vi "UHR-Fleezers Control (host) - 11.9c.vi"() -> ()   [LabVIEW 2014] (continued)
          tunnel: [w2795] -> w2786
          tunnel: w2792 -> [w2812]
          tunnel: w2791 -> [w2811]
          tunnel: [w2809] -> w2790
          tunnel: w2789 -> [w2810]
          tunnel: [w2808] -> w2788
          tunnel: [w2807] -> w2787
          tunnel: w2786 -> [w2807]
          tunnel: w2790 -> [w2816]
          tunnel: w2788 -> [w2815]
          tunnel: w2787 -> [w2814]
          frame #0 {
            n1958 = call "Read Stage Position.vi"("error in"=w2805, "VISA resource name in"=w2797) -> ("Current Position"=w2795:cluster{dbl, dbl, dbl}, "error out"=w2798:errorcluster, "VISA resource name out"=w2796:refnum<visa-resource-name>)  [unwired: 1 out]
            "Current Position" <- w2795
            n1959 = local write "Stage Control Serial Error"(w2798) -> ()
            n1960 = Unbundle(w2795) -> (w2802:dbl, w2804:dbl, w2800:dbl)
            n1961 = Add(x=w2804, y="Y change (mm)") -> (x+y=w2801:dbl)
            n1962 = Bundle(w2802, w2801, w2800) -> (w2799:cluster{dbl, dbl, dbl})  [unwired: 1 in]
          }
          frame #1 {
            # "move to new position and start saving"
            n1963 = local write "Stage Moving"(TRUE ("Stage Moving")) -> ()
            n1964 = local write "Start Saving"(TRUE ("Start Saving")) -> ()
            n1965 = call "Set Stage Position.vi"("Position"=w2812, "error in"=w2811, "VISA resource name in"=w2810) -> ("error out"=w2808:errorcluster, "VISA resource name out"=w2809:refnum<visa-resource-name>)  [unwired: 1 out]
          }
          frame #2 {
            # "go back to start"
            n1966 = call "Set Stage Position.vi"("Position"=w2814, "error in"=w2815, "VISA resource name in"=w2816) -> ()  [unwired: 3 out]
          }
          frame #3 {
            # "stop saving"
            n1967 = local write "Stop Saving"(TRUE ("Stop Saving")) -> ()
            n1968 = local write "Stage Moving"(FALSE ("Stage Moving")) -> ()
          }
        }
      }
      event "Move to Position 1", "Move to Position 2", "Move to Position 3", "Move to Position 4", "Move to Position 5", "Lower Ch. Cap.": Value Change {
        n1969 = event-data() -> ()  [unwired: 1 in, 5 out]
        n1970 = Or(x="Move to Position 5", y="Lower Ch. Cap.") -> (x .or. y?=w2822:bool)
        n1971 = Build Array("Move to Position 1", "Move to Position 2", "Move to Position 3", "Move to Position 4", w2822) -> (w2825:bool[])
        n1972 = Boolean Array To Number(Boolean array=w2825) -> (number=w2824:u32)
        n1973 = Logarithm Base 2(1:w2824) -> (0:w2823:dbl)
        n1974 = flat-sequence {
          tunnel: w2823 -> [w2834]
          tunnel: w2820 -> [w2832]
          tunnel: w2819 -> [w2831]
          frame #0 {
            n1975 = local read "Saved Stage Positions"() -> (w2842:dbl[][])
            n1976 = Array Subset(array=w2842, index (row)=w2834, length (row)=1 ("length"), index (col)=1 ("index"), length (col)=3 ("length")) -> (w2839:dbl[][])
            n1977 = Reshape Array(w2839, 3 ("dimension size")) -> (w2837:dbl[])
            n1978 = Array To Cluster(array=w2837) -> (cluster=w2836:cluster{"[0]":dbl, "[1]":dbl, "[2]":dbl})
            n1979 = call "Set Stage Position.vi"("Position"=w2836, "error in"=w2831, "VISA resource name in"=w2832) -> ("error out"=w2835:errorcluster)  [unwired: 2 out]
            n1980 = local write "Stage Moving"(TRUE ("Stage Moving")) -> ()
            n1981 = local write "Stage Control Serial Error"(w2835) -> ()
          }
          frame #1 {
            n1982 = local write "Stage Moving"(FALSE ("Stage Moving")) -> ()
            n1983 = call <vilib>:"Beep.vi"() -> ()  [unwired: 3 in, 9 out]
          }
        }
      }
      event "Set Current\nPos to 0,0,0": Value Change {
        # "DH is \"Define Home\""
        n1984 = event-data() -> ()  [unwired: 1 in, 6 out]
        n1985 = local write "Set Current\nPos to 0,0,0"(FALSE ("Set Current\nPos to 0,0,0")) -> ()
        n1986 = Concatenate Strings("1DH" ("string"), ";" ("string"), "2DH" ("string"), ";" ("string"), "3DH" ("string"), "\r") -> (w2850:string)
        n1987 = call-poly "VISA Configure Serial Port"("VISA resource name"=w2855, "baud rate (9600)"=u32 19200, "error in (no error)"=w2854) -> ("VISA resource name out"=w2852:refnum<visa-resource-name>, "error out"=w2851:errorcluster)  [unwired: 11 in]
        n1988 = VISA Write(VISA resource name=w2852, write buffer=w2850, error in (no error)=w2851) -> (error out=w2845:errorcluster)  [unwired: 2 out]
        n1989 = local write "Stage Control Serial Error"(w2845) -> ()
      }
      event "Got ADig bead": Value Change {
        n1990 = event-data() -> ()  [unwired: 1 in, 5 out]
        n1991 = flat-sequence {
          frame #0 {
            n1992 = local read "Cap 1 Samp Flow ON"() -> (w2860:bool)
            n1993 = case shown="True" w2860 {
              frame False {
              }
              frame True {
                n1994 = property on="Sample Channel\nFlow" class="Bool (strict)"("Val(Sgnl)"=TRUE ("Value (Signaling)")) -> ()  [unwired: 2 in, 2 out]
              }
            }
          }
          frame #1 {
            n1995 = property on="Inject Pump 3" class="Bool (strict)"("Val(Sgnl)"=FALSE ("Value (Signaling)")) -> ()  [unwired: 2 in, 2 out]
            n1996 = local write "Target"(FALSE ("Target")) -> ()
          }
          frame #2 {
            n1997 = property on="Move Cap. 1 (DNA Bottom)" class="Bool (strict)"("Val(Sgnl)"=TRUE ("Value (Signaling)")) -> ()  [unwired: 2 in, 2 out]
          }
        }
      }
      event "Force FB Script": Value Change {
        n1998 = event-data() -> ()  [unwired: 1 in, 5 out]
        n1999 = local write "Force FB Script"(FALSE ("Force FB Data\nScript")) -> ()
        n2000 = flat-sequence {
          tunnel: w2871 -> [w2875]
          tunnel: w2872 -> [w2876]
          tunnel: [w2876] -> w2867
          tunnel: [w2875] -> w2866
          tunnel: w2867 -> [w2879]
          tunnel: w2866 -> [w2878]
          tunnel: ["Trap Trig Fl."] -> w2868
          tunnel: [w2921] -> w2869
          tunnel: w2868 -> [w2921]
          tunnel: [w2925] -> w2870
          tunnel: w2869 -> [w2925]
          tunnel: w2870 -> [w2927]
          frame #0 {
            n2001 = property on="Trap D (MHz)" class="DigNum (strict)"("Val(Sgnl)"="Trap D Before Moving") -> ()  [unwired: 2 in, 2 out]
          }
          frame #1 {
            n2002 = local read "Saved Stage Positions"() -> (w2881:dbl[][])
            n2003 = local write "FB Trap Pos Offset"(0.0 ("FB Trap Pos Offset")) -> ()
            n2004 = property on="Trap Pos. FB Offset Factor" class="DigNum (strict)"("Val(Sgnl)"=i64 0 ("Value (Signaling)")) -> ()  [unwired: 2 in, 2 out]
            n2005 = local write "Stage Moving"(TRUE ("Stage Moving")) -> ()
            n2006 = call "move to saved stage position.vi"("error in"=w2878, "Stage VISA resource name in"=w2879, "Position"="Stage Position To Establish FB", "Saved Stage Positions"=w2881) -> ("error out"=w2877:errorcluster)  [unwired: 1 out]
            n2007 = local write "Stage Control Serial Error"(w2877) -> ()
          }
          frame #2 {
            n2008 = call <vilib>:"Beep.vi"("duration (msec)"=u32 100, "frequency (Hz)"=u32 20) -> ()  [unwired: 1 in, 9 out]
            n2009 = local write "Stage Moving"(FALSE ("Stage Moving")) -> ()
            n2010 = property on="Tab Control 2" class="TabCtl (strict)"("Val(Sgnl)"=T6."Feedback on Trap Position" ("Value (Signaling)")) -> ()  [unwired: 2 in, 2 out]
            n2011 = stacked-sequence {
              frame #0 {
                n2012 = Multiply(x="Wait (s)", y=u32 1000 ("milliseconds to wait")) -> (x*y=w2890:u32)
                n2013 = property on="Trap D (MHz)" class="DigNum (strict)"("Val(Sgnl)"="Starting Trap D (MHz)") -> ()  [unwired: 2 in, 2 out]
                n2014 = Wait (ms)(milliseconds to wait=w2890) -> ()  [unwired: 1 out]
              }
              frame #1 {
                n2015 = property on="Set Reading to\nSetpoint" class="Bool (strict)"("Val(Sgnl)"=TRUE ("Value (Signaling)")) -> ()  [unwired: 2 in, 2 out]
              }
            }
            n2016 = property on="Tab Control" class="TabCtl (strict)"("Val(Sgnl)"=T4."Trap Control (RF)" ("Value (Signaling)")) -> ()  [unwired: 2 in, 2 out]
          }
          frame #3 {
            n2017 = Wait (ms)(milliseconds to wait=u32 500) -> ()  [unwired: 1 out]
          }
          frame #4 {
            n2018 = property on="Trap Pos. FB ON" class="Bool (strict)"("Val(Sgnl)"=TRUE ("Value (Signaling)")) -> ()  [unwired: 2 in, 2 out]
            n2019 = Wait (ms)(milliseconds to wait=u32 250) -> ()  [unwired: 1 out]
          }
          frame #5 {
            n2020 = case shown="\"1\"" "Remove Action Offset Dropdown" {
              tunnel: TRUE ("Value (Signaling)") -> [w2902 w2910 w2918]
              frame "1" {
                n2021 = flat-sequence {
                  tunnel: w2902 -> [w2909]
                  frame #0 {
                    n2022 = local read "factor"() -> (w2904:dbl)
                    n2023 = Greater Than 0?(x=w2904) -> (x > 0?=w2908:bool)
                    n2024 = Select(t=1.0, s=w2908, f=-1.0) -> (s? t:f=w2905:dbl)
                    n2025 = Multiply(x=w2905, y=w2904) -> (x*y=w2903:dbl)
                    n2026 = local write "factor"(w2903) -> ()
                  }
                  frame #1 {
                    n2027 = property on="Remove Offset to factor" class="Bool (strict)"("Val(Sgnl)"=w2909) -> ()  [unwired: 2 in, 2 out]
                  }
                }
              }
              frame "2" {
                n2028 = flat-sequence {
                  tunnel: w2910 -> [w2917]
                  frame #0 {
                    n2029 = local read "factor"() -> (w2911:dbl)
                    n2030 = Greater Than 0?(x=w2911) -> (x > 0?=w2916:bool)
                    n2031 = Select(t=-1.0, s=w2916, f=1.0) -> (s? t:f=w2914:dbl)
                    n2032 = Multiply(x=w2911, y=w2914) -> (x*y=w2913:dbl)
                    n2033 = local write "factor"(w2913) -> ()
                  }
                  frame #1 {
                    n2034 = property on="Remove Offset to factor" class="Bool (strict)"("Val(Sgnl)"=w2917) -> ()  [unwired: 2 in, 2 out]
                  }
                }
              }
              frame "0", Default {
                n2035 = property on="Remove Action Offset" class="Bool (strict)"("Val(Sgnl)"=w2918) -> ()  [unwired: 2 in, 2 out]
              }
            }
            n2036 = case shown="False" "Trap Trig Fl." {
              frame False {
                n2037 = case shown="True" "Green ON after FB ON?" {
                  selector: "Green ON after FB ON?" -> [_ w2920]
                  frame False {
                  }
                  frame True {
                    n2038 = property on="Green ON/Interlacing" class="Bool (strict)"("Val(Sgnl)"=w2920) -> ()  [unwired: 2 in, 2 out]
                  }
                }
              }
              frame True {
              }
            }
            n2039 = Wait (ms)(milliseconds to wait=u32 250) -> ()  [unwired: 1 out]
          }
          frame #6 {
            n2040 = property on="Start Saving" class="Bool (strict)"("Val(Sgnl)"=TRUE ("Value (Signaling)")) -> ()  [unwired: 2 in, 2 out]
            n2041 = Wait (ms)(milliseconds to wait=u32 5000) -> ()  [unwired: 1 out]
          }
          frame #7 {
            w2924 = TRUE ("Value (Signaling)")
            n2042 = property on="Rem fb disp offset" class="Bool (strict)"("Val(Sgnl)"=w2924) -> ()  [unwired: 2 in, 2 out]
            n2043 = property on="Remove Offset" class="Bool (strict)"("Val(Sgnl)"=w2924) -> ()  [unwired: 2 in, 2 out]
            n2044 = Wait (ms)(milliseconds to wait=u32 100) -> ()  [unwired: 1 out]
          }
          frame #8 {
            n2045 = case shown="True" w2927 {
              frame False {
              }
              frame True {
                n2046 = local write "Trap Trig. Fl."(TRUE ("Value (Signaling)")) -> ()
              }
            }
          }
          frame #9 {
            n2047 = local read "Tether"() -> (w2930:bool)
            n2048 = And(x="Start dipping after?", y=w2930) -> (x .and. y?=w2929:bool)
            n2049 = case shown="True" w2929 {
              frame False {
              }
              frame True {
                n2050 = flat-sequence {
                  frame #0 {
                    n2051 = Multiply(x="Delay before dipping (s)", y=1000.0) -> (x*y=w2933:dbl)
                    n2052 = Wait (ms)(milliseconds to wait=w2933) -> ()  [unwired: 1 out]
                  }
                  frame #1 {
                    n2053 = property on="Dip for Protein" class="Bool (strict)"("Val(Sgnl)"=TRUE ("Value (Signaling)")) -> ()  [unwired: 2 in, 2 out]
                    n2054 = local write "Scripts"(T30."Dipping") -> ()
                  }
                }
              }
            }
          }
        }
      }
      event "Rupture Script": Value Change {
        n2055 = event-data() -> ()  [unwired: 1 in, 5 out]
        n2056 = local write "Rupture Script"(FALSE ("Rupture Script")) -> ()
        n2057 = flat-sequence {
          frame #0 {
            w2939 = TRUE
            w2944 = FALSE
            # "Number 6 for now is the\nrupture-experiment\nparameters."
            n2058 = local read "Starting Trap D (MHz)"() -> (w2945:dbl)
            n2059 = local write "Restart DMA? (AOD)"(w2944) -> ()
            n2060 = Replace Array Subset(array=u32[] [0] ("Index Values"), new element=6, index=0) -> (w2940:u32[])
            n2061 = local write "Save scans"(w2944) -> ()
            n2062 = property on="Trap D (MHz)" class="DigNum (strict)"("Val(Sgnl)"=w2945) -> ()  [unwired: 2 in, 2 out]
            n2063 = property on="Saved AOD Raster Scan Parameter Sets" class="Arr (strict)"("Index Values"=w2940) -> ()  [unwired: 2 in, 2 out]
            n2064 = property on="Start Saving" class="Bool (strict)"("Val(Sgnl)"=w2939) -> ()  [unwired: 2 in, 2 out]
            n2065 = property on="Green ON/Interlacing" class="Bool (strict)"("Val(Sgnl)"=w2939) -> ()  [unwired: 2 in, 2 out]
          }
          frame #1 {
            n2066 = property on="Load parameters" class="Bool (strict)"("Val(Sgnl)"=TRUE ("Value (Signaling)")) -> ()  [unwired: 2 in, 2 out]
          }
        }
      }
      event "Fixed Traps Script": Value Change {
        n2067 = event-data() -> ()  [unwired: 1 in, 5 out]
        n2068 = local write "Fixed Traps Script"(FALSE ("Fixed Traps Data\nScript")) -> ()
        n2069 = flat-sequence {
          frame #0 {
            n2070 = case shown="True" "Green ON" {
              frame False {
              }
              frame True {
                n2071 = property on="Green ON/Interlacing" class="Bool (strict)"("Val(Sgnl)"=TRUE) -> ()  [unwired: 2 in, 2 out]
              }
            }
            n2072 = local write "Offset (nm)"(0.0 ("Offset (nm)")) -> ()
            n2073 = property on="Sample Channel\nFlow" class="Bool (strict)"("Val(Sgnl)"=FALSE ("Value (Signaling)")) -> ()  [unwired: 2 in, 2 out]
            n2074 = property on="Trap D (MHz)" class="DigNum (strict)"("Val(Sgnl)"="Fixed Traps Trap Delta (MHz)") -> ()  [unwired: 2 in, 2 out]
          }
          frame #1 {
            n2075 = Wait (ms)(milliseconds to wait=u32 1000) -> ()  [unwired: 1 out]
          }
          frame #2 {
            n2076 = local write "Start Saving"(TRUE ("Start Saving")) -> ()
          }
          frame #3 {
            n2077 = local read "Bead Sep. Int. Time (s)"() -> (w2955:dbl)
            n2078 = Multiply(x=w2955, y=1000.0) -> (x*y=w2957:dbl)
            n2079 = Wait (ms)(milliseconds to wait=w2957) -> ()  [unwired: 1 out]
          }
          frame #4 {
            n2080 = property on="Remove Offset" class="Bool (strict)"("Val(Sgnl)"=TRUE ("Value (Signaling)")) -> ()  [unwired: 2 in, 2 out]
          }
          frame #5 {
            n2081 = property on="Dip for Protein" class="Bool (strict)"("Val(Sgnl)"="Start dipping after?") -> ()  [unwired: 2 in, 2 out]
          }
        }
      }
      event "Got DNA bead": Value Change {
        n2082 = event-data() -> ()  [unwired: 1 in, 5 out]
        n2083 = flat-sequence {
          frame #0 {
            n2084 = local read "Daq spot flow on"() -> (w2962:bool)
            n2085 = case shown="True" w2962 {
              frame False {
              }
              frame True {
                n2086 = property on="Sample Channel\nFlow" class="Bool (strict)"("Val(Sgnl)"=TRUE ("Value (Signaling)")) -> ()  [unwired: 2 in, 2 out]
              }
            }
            n2087 = property on="Got DNA bead" class="Bool"("Key Focus"=FALSE) -> ()  [unwired: 2 in, 2 out]
          }
          frame #1 {
            n2088 = property on="Inject Pump 1" class="Bool (strict)"("Val(Sgnl)"=FALSE ("Value (Signaling)")) -> ()  [unwired: 2 in, 2 out]
          }
          frame #2 {
            n2089 = property on="Cal/Data Acq. Spot" class="Bool (strict)"("Val(Sgnl)"=TRUE ("Value (Signaling)")) -> ()  [unwired: 2 in, 2 out]
          }
        }
      }
      event "Take Stepping Data": Value Change {
        n2090 = event-data() -> ()  [unwired: 1 in, 5 out]
        n2091 = local read "Save ave N"() -> (w2974:dbl)
        n2092 = flat-sequence {
          tunnel: w2974 -> [w2976]
          tunnel: [w2976] -> w2969
          tunnel: [w2978] -> w2970
          tunnel: w2969 -> [w2978]
          tunnel: [w2980] -> w2971
          tunnel: w2970 -> [w2980]
          tunnel: [w2983] -> w2972
          tunnel: w2971 -> [w2983]
          tunnel: [w2985] -> w2973
          tunnel: w2972 -> [w2985]
          tunnel: [w2987] -> w2967
          tunnel: w2973 -> [w2987]
          tunnel: w2967 -> [w2990]
          tunnel: [w2990] -> w2966
          tunnel: w2966 -> [w2991]
          tunnel: [w2991] -> w2968
          tunnel: w2968 -> [w2997]
          frame #0 {
            n2093 = property on="Save ave N" class="DigNum (strict)"("Val(Sgnl)"="Save ave factor") -> ()  [unwired: 2 in, 2 out]
          }
          frame #1 {
            n2094 = Wait (ms)(milliseconds to wait=u32 100) -> ()  [unwired: 1 out]
          }
          frame #2 {
            n2095 = local read "Offset 2 Start (MHz)"() -> (w2982:dbl)
            n2096 = property on="Saved AOD Raster Scan Parameter Sets" class="Arr (strict)"("Index Values"=u32[] [2]) -> ()  [unwired: 2 in, 2 out]
            n2097 = property on="Trap D (MHz)" class="DigNum (strict)"("Val(Sgnl)"=w2982) -> ()  [unwired: 2 in, 2 out]
          }
          frame #3 {
            n2098 = property on="Load parameters" class="Bool (strict)"("Val(Sgnl)"=TRUE ("Value (Signaling)")) -> ()  [unwired: 2 in, 2 out]
          }
          frame #4 {
            n2099 = Wait (ms)(milliseconds to wait=u32 100) -> ()  [unwired: 1 out]
          }
          frame #5 {
            n2100 = property on="Trap Raster Scan" class="Bool (strict)"("Val(Sgnl)"=TRUE ("Value (Signaling)")) -> ()  [unwired: 2 in, 2 out]
          }
          frame #6 {
            n2101 = Wait (ms)(milliseconds to wait=u32 1000) -> ()  [unwired: 1 out]
          }
          frame #7 {
            n2102 = while {
              stop <- w2994 stop-if-true
              n2103 = local read "Raster Scanning..."() -> (w2996:bool)
              n2104 = local read "Saving..."() -> (w2995:bool)
              n2105 = Not(x=w2995) -> (.not. x?=w2992:bool)
              n2106 = Not(x=w2996) -> (.not. x?=w2993:bool)
              n2107 = And(x=w2993, y=w2992) -> (x .and. y?=w2994:bool)
            }
          }
          frame #8 {
            n2108 = property on="Save ave N" class="DigNum (strict)"("Val(Sgnl)"=w2997) -> ()  [unwired: 2 in, 2 out]
          }
        }
      }
      event "Step Size (nm)": Value Change {
        n2109 = event-data() -> ()  [unwired: 1 in, 5 out]
        n2110 = flat-sequence {
          frame #0 {
            n2111 = property on="Saved AOD Raster Scan Parameter Sets" class="Arr (strict)"("Index Values"=u32[] [1]) -> ()  [unwired: 2 in, 2 out]
          }
          frame #1 {
            n2112 = Multiply(x="N Steps", y="Step Size (nm)") -> (x*y=w2999:dbl)
            n2113 = property on="Scan Speed AOD (nm/s) 2" class="DigNum (strict)"("Value"="Step Size (nm)") -> ()  [unwired: 2 in, 2 out]
            n2114 = property on="Step Size AOD (nm) 2" class="DigNum (strict)"("Value"="Step Size (nm)") -> ()  [unwired: 2 in, 2 out]
            n2115 = property on="Scan Range AOD (nm) 2" class="DigNum (strict)"("Value"=w2999) -> ()  [unwired: 2 in, 2 out]
          }
        }
      }
      event "Take Detection Laser\nImage": Value Change {
        n2116 = event-data() -> ()  [unwired: 1 in, 5 out]
        n2117 = flat-sequence {
          tunnel: [w3027] -> w3017
          tunnel: [w3026] -> w3010
          tunnel: [w3025] -> w3002
          tunnel: [w3030] -> w3018
          tunnel: w3017 -> [w3030]
          tunnel: [w3029] -> w3011
          tunnel: w3010 -> [w3029]
          tunnel: [w3028] -> w3003
          tunnel: w3002 -> [w3028]
          tunnel: [w3034] -> w3019
          tunnel: w3018 -> [w3034]
          tunnel: [w3033] -> w3012
          tunnel: w3011 -> [w3033]
          tunnel: [w3032] -> w3004
          tunnel: w3003 -> [w3032]
          tunnel: [w3040] -> w3020
          tunnel: w3019 -> [w3040]
          tunnel: [w3039] -> w3013
          tunnel: w3012 -> [w3039]
          tunnel: [w3038] -> w3005
          tunnel: w3004 -> [w3038]
          tunnel: [w3044] -> w3021
          tunnel: w3020 -> [w3044]
          tunnel: [w3043] -> w3014
          tunnel: w3013 -> [w3043]
          tunnel: [w3042] -> w3006
          tunnel: w3005 -> [w3042]
          tunnel: [w3048] -> w3022
          tunnel: w3021 -> [w3048]
          tunnel: [w3047] -> w3015
          tunnel: w3014 -> [w3047]
          tunnel: [w3046] -> w3007
          tunnel: w3006 -> [w3046]
          tunnel: [w3052] -> w3023
          tunnel: w3022 -> [w3052]
          tunnel: [w3051] -> w3016
          tunnel: w3015 -> [w3051]
          tunnel: [w3050] -> w3008
          tunnel: w3007 -> [w3050]
          tunnel: w3023 -> [w3058]
          tunnel: w3016 -> [w3057]
          tunnel: [w3055] -> w3009
          tunnel: w3008 -> [w3055]
          tunnel: w3009 -> [w3059]
          frame #0 {
            n2118 = local read "Laser interlacing mode (all lasers)"() -> (w3026:enum32{"Laser ON", "Laser OFF", "Interlace"})
            n2119 = local read "Green ON/Interlacing"() -> (w3027:bool)
            n2120 = local read "Green FB On/Off"() -> (w3025:bool)
          }
          frame #1 {
            n2121 = property on="Green FB On/Off" class="Bool (strict)"("Val(Sgnl)"=FALSE ("Value (Signaling)")) -> ()  [unwired: 2 in, 2 out]
          }
          frame #2 {
            n2122 = property on="Green ON/Interlacing" class="Bool (strict)"("Val(Sgnl)"=TRUE ("Value (Signaling)")) -> ()  [unwired: 2 in, 2 out]
            n2123 = property on="Flip Green Filter" class="Bool (strict)"("Val(Sgnl)"=TRUE ("Value (Signaling)")) -> ()  [unwired: 2 in, 2 out]
            n2124 = property on="Laser interlacing mode (all lasers)" class="RadioBtnsControl (strict)"("Val(Sgnl)"=enum32{"Laser ON", "Laser OFF", "Interlace"}."Laser ON" ("Value (Signaling)")) -> ()  [unwired: 2 in, 2 out]
          }
          frame #3 {
            n2125 = Wait (ms)(milliseconds to wait=u32 500) -> ()  [unwired: 1 out]
          }
          frame #4 {
            n2126 = property on="Confocal\nImage" class="Bool (strict)"("Val(Sgnl)"=TRUE ("Value (Signaling)")) -> ()  [unwired: 2 in, 2 out]
          }
          frame #5 {
            n2127 = Wait (ms)(milliseconds to wait=u32 2000) -> ()  [unwired: 1 out]
          }
          frame #6 {
            n2128 = while {
              stop <- w3053 stop-if-true
              n2129 = local read "Saving..."() -> (w3054:bool)
              n2130 = Not(x=w3054) -> (.not. x?=w3053:bool)
            }
          }
          frame #7 {
            n2131 = property on="Flip Green Filter" class="Bool (strict)"("Val(Sgnl)"=TRUE ("Value (Signaling)")) -> ()  [unwired: 2 in, 2 out]
            n2132 = property on="Green ON/Interlacing" class="Bool (strict)"("Val(Sgnl)"=w3058) -> ()  [unwired: 2 in, 2 out]
            n2133 = property on="Laser interlacing mode (all lasers)" class="RadioBtnsControl (strict)"("Val(Sgnl)"=w3057) -> ()  [unwired: 2 in, 2 out]
          }
          frame #8 {
            n2134 = property on="Green FB On/Off" class="Bool (strict)"("Val(Sgnl)"=w3059) -> ()  [unwired: 2 in, 2 out]
          }
        }
      }
      event "Stop All": Value Change {
        n2135 = event-data() -> ()  [unwired: 1 in, 5 out]
        n2136 = local read "Stop All"() -> (w3060:bool)
      }
    }
    n2137 = node-c288() -> ()  [unwired: 1 in, 1 out]
  }
  n2138 = node-c288() -> (w122:T22)  [unwired: 4 out]
  n2139 = timed-loop "Mouse control: trap position (AOM deflection), set confocal spot from image" {
    tunnel: [w3062] -> w207
    tunnel: w32 -> [w3061]
    timing: w122 -> [_]
    timing-out: [_] -> w121
    stop <- w3062 stop-if-true
    n2140 = node-c288() -> ()  [unwired: 2 out]
    n2141 = event shown="[0] \"Pane\": Mouse Down" {
      selector: _ -> [_ _]
      dyn-events: _ -> [_ _]
      timeout: _ -> [_ _]
      tunnel: w3061 -> [w3065 _]
      event Mouse Down {
        n2142 = event-data() -> ("Time"=w3067:u32, "Coords"=w3066:T7, "Button"=w3068:u16)  [unwired: 6 out]
        n2143 = case shown="1" w3068 {
          tunnel: w3067 -> [_ _ w3207]
          tunnel: w3066 -> [_ w3073 w3205]
          tunnel: w3065 -> [_ _ w3203]
          frame 0, Default {
          }
          frame 1 {
            n2144 = property on="APD 2" class="ImageControl"() -> ("Displayed Image Position"=w3087:cluster{"Left":i32, "Top":i32})  [unwired: 2 in, 2 out]
            n2145 = control-ref of="Primary Video Display"() -> (w3080:refnum<vi>)
            n2146 = property on="APD 1" class="ImageControl"() -> ("Displayed Image Position"=w3116:cluster{"Left":i32, "Top":i32})  [unwired: 2 in, 2 out]
            n2147 = property on="Detection Laser X" class="ImageControl"() -> ("Displayed Image Position"=w3113:cluster{"Left":i32, "Top":i32})  [unwired: 2 in, 2 out]
            n2148 = property on="Detection Laser Y" class="ImageControl"() -> ("Displayed Image Position"=w3112:cluster{"Left":i32, "Top":i32})  [unwired: 2 in, 2 out]
            n2149 = property on="APD 2" class="ImageControl"() -> ("Displayed Image Size"=w3086:cluster{"Width":u32, "Height":u32})  [unwired: 2 in, 2 out]
            n2150 = property on="APD 1" class="ImageControl"() -> ("Displayed Image Size"=w3114:cluster{"Width":u32, "Height":u32})  [unwired: 2 in, 2 out]
            n2151 = property on="Detection Laser X" class="ImageControl"() -> ("Displayed Image Size"=w3115:cluster{"Width":u32, "Height":u32})  [unwired: 2 in, 2 out]
            n2152 = property on="Detection Laser Y" class="ImageControl"() -> ("Displayed Image Size"=w3111:cluster{"Width":u32, "Height":u32})  [unwired: 2 in, 2 out]
            n2153 = property class="ImageControl"(reference=w3080) -> ("Displayed Image Position"=w3078:cluster{"Left":i32, "Top":i32})  [unwired: 1 in, 2 out]
            n2154 = property class="ImageControl"(reference=w3080) -> ("Displayed Image Size"=w3079:cluster{"Width":u32, "Height":u32})  [unwired: 1 in, 2 out]
            n2155 = Unbundle By Name(w3086) -> ("Width"=w3083:u32, "Height"=w3082:u32)
            n2156 = Unbundle By Name(w3087) -> ("Left"=w3085:i32, "Top"=w3084:i32)
            n2157 = Unbundle By Name(w3114) -> ("Width"=w3108:u32, "Height"=w3107:u32)
            n2158 = Unbundle By Name(w3115) -> ("Width"=w3104:u32, "Height"=w3103:u32)
            n2159 = Unbundle By Name(w3111) -> ("Width"=w3100:u32, "Height"=w3099:u32)
            n2160 = Unbundle By Name(w3116) -> ("Left"=w3110:i32, "Top"=w3109:i32)
            n2161 = Unbundle By Name(w3113) -> ("Left"=w3106:i32, "Top"=w3105:i32)
            n2162 = Unbundle By Name(w3112) -> ("Left"=w3102:i32, "Top"=w3101:i32)
            n2163 = Bundle("Left"=w3085, "Top"=w3084, "Width"=w3083, "Height"=w3082) -> (w3081:T31)  [unwired: 1 in]
            n2164 = Bundle("Left"=w3110, "Top"=w3109, "Width"=w3108, "Height"=w3107) -> (w3098:T31)  [unwired: 1 in]
            n2165 = Bundle("Left"=w3106, "Top"=w3105, "Width"=w3104, "Height"=w3103) -> (w3097:T31)  [unwired: 1 in]
            n2166 = Bundle("Left"=w3102, "Top"=w3101, "Width"=w3100, "Height"=w3099) -> (w3096:T31)  [unwired: 1 in]
            n2167 = Unbundle By Name(w3079) -> ("Width"=w3075:u32, "Height"=w3074:u32)
            n2168 = Unbundle By Name(w3078) -> ("Left"=w3077:i32, "Top"=w3076:i32)
            n2169 = Build Cluster Array(w3081, w3098, w3097, w3096) -> (w3095:T32)
            n2170 = Bundle("Left"=w3077, "Top"=w3076, "Width"=w3075, "Height"=w3074) -> (w3070:T31)  [unwired: 1 in]
            n2171 = for {
              tunnel: w3073 -> [w3149]
              tunnel: w3095 -> [w3150] mode=indexing
              shift-right: [w3147] -> w3093
              shift-left: TRUE -> [w3148]
              shift-right: [w3146] -> w3091
              shift-left: _ -> [w3142]
              shift-right: [w3145] -> w3090
              shift-left: _ -> [w3141]
              shift-right: [w3144] -> w3089
              shift-left: _ -> [w3140]
              shift-right: [w3143] -> w3088
              shift-left: _ -> [w3139]
              n2172 = case shown="True" w3148 {
                selector: w3148 -> [w3155 _]
                tunnel: w3150 -> [_ w3164]
                tunnel: w3149 -> [_ w3162]
                tunnel: [w3155 w3160] -> w3147
                tunnel: [w3154 w3159] -> w3146
                tunnel: [w3153 w3158] -> w3145
                tunnel: [w3152 w3157] -> w3144
                tunnel: [w3151 w3156] -> w3143
                tunnel: w3142 -> [w3154 _]
                tunnel: w3141 -> [w3153 _]
                tunnel: w3140 -> [w3152 _]
                tunnel: w3139 -> [w3151 _]
                frame False {
                }
                frame True {
                  n2173 = Unbundle(w3164) -> (w3163:T31)
                  n2174 = call "isclickinwindow.vi"("Image Param"=w3163, "Point32"=w3162) -> ("4 Y"=w3156:i32, "3 Height"=w3157:i32, "2 X"=w3158:i32, "1 Width"=w3159:i32, "In image?"=w3161:bool)  [unwired: 1 in]
                  n2175 = Not(x=w3161) -> (.not. x?=w3160:bool)
                }
              }
            }
            n2176 = call "isclickinwindow.vi"("Image Param"=w3070, "Point32"=w3073) -> ("4 Y"=w3071:i32, "2 X"=w3072:i32, "In image?"=w3069:bool)  [unwired: 1 in, 2 out]
            n2177 = case shown="True" w3069 {
              tunnel: w3072 -> [_ w3120]
              tunnel: w3071 -> [_ w3123]
              frame False {
              }
              frame True {
                w3132 = 2
                n2178 = Subtract(x=480, y=w3123) -> (x-y=w3122:i32)
                n2179 = Unbundle("Target size") -> ("Width"=w3133:dbl, "Height"=w3131:dbl)
                n2180 = Subtract(x=w3120, y=2) -> (x-y=w3119:i32)
                n2181 = Divide(x=w3131, y=w3132) -> (x/y=w3129:dbl)
                n2182 = Divide(x=w3133, y=w3132) -> (x/y=w3130:dbl)
                n2183 = Subtract(x=w3119, y=w3130) -> (x-y=w3128:dbl)
                n2184 = Add(x=w3119, y=w3130) -> (x+y=w3126:dbl)
                n2185 = Subtract(x=w3122, y=w3129) -> (x-y=w3127:dbl)
                n2186 = Add(x=w3122, y=w3129) -> (x+y=w3125:dbl)
                n2187 = Bundle(w3119, w3122) -> (w3135:cluster{i32, i32})  [unwired: 1 in]
                n2188 = Bundle(w3128, w3127, w3126, w3125) -> (w3117:cluster{dbl, dbl, dbl, dbl})  [unwired: 1 in]
                n2189 = case shown="True" "Set target" {
                  tunnel: w3135 -> [_ w3138]
                  tunnel: w3117 -> [_ w3136]
                  frame False {
                  }
                  frame True {
                    n2190 = local write "Target coordinates"(w3136) -> ()
                    n2191 = local write "Set target"(FALSE ("Set target")) -> ()
                    "Video coordinates" <- w3138
                  }
                }
              }
            }
            n2192 = Not(x=w3093) -> (.not. x?=w3092:bool)
            n2193 = case shown="True" w3092 {
              tunnel: w3090 -> [_ w3178]
              tunnel: w3088 -> [_ w3177]
              tunnel: w3091 -> [_ w3176]
              tunnel: w3089 -> [_ w3175]
              frame False {
              }
              frame True {
                w3165 = FALSE ("Get Point")
                n2194 = local read "Scan lines (y)"() -> (w3180:u64)
                n2195 = disable-structure shown="Disabled" {
                  frame Disabled {
                  }
                  frame Enabled {
                  }
                }
                n2196 = local read "Actual MCL Inc (V)"() -> (w3174:dbl)
                n2197 = local read "Scan steps (MCL)"() -> (w3179:u64)
                n2198 = Divide "Y Pix/step"(x=w3175, y=w3180) -> (x/y=w3187:dbl)
                n2199 = Divide "Y V/pix"(x=w3174, y=w3187) -> (x/y=w3186:dbl)
                n2200 = Divide "Y half step offset"(x=w3174, y=2.0) -> (x/y=w3188:dbl)
                n2201 = Divide "X pix/step"(x=w3176, y=w3179) -> (x/y=w3185:dbl)
                n2202 = Negate(x=w3188) -> (-x=w3189:dbl)
                n2203 = local read "Initial Y"() -> (w3195:dbl)
                n2204 = Multiply(x=w3177, y=w3186) -> (x*y=w3196:dbl)
                n2205 = Divide "X half step offset"(x=w3174, y=2.0) -> (x/y=w3182:dbl)
                n2206 = Divide "X V/pix"(x=w3174, y=w3185) -> (x/y=w3184:dbl)
                n2207 = Multiply(x=w3174, y=w3179) -> (x*y=w3191:dbl)
                n2208 = Compound Arithmetic op=ADD(w3189, w3196, w3195) -> (w3166:dbl)
                "Pointer Y (V)" <- w3166
                n2209 = Multiply(x=w3184, y=w3178) -> (x*y=w3193:dbl)
                n2210 = Negate(x=w3182) -> (-x=w3181:dbl)
                n2211 = local read "Initial X"() -> (w3194:dbl)
                n2212 = Negate(x=w3193) -> (-x=w3192:dbl)
                n2213 = Compound Arithmetic op=ADD(w3181, w3191, w3194, w3192) -> (w3167:dbl)
                "Pointer X (V)" <- w3167
                n2214 = case shown="True" "Set High F Confocal Spot (X-Y)" {
                  tunnel: w3167 -> [_ w3197]
                  tunnel: w3166 -> [_ w3198]
                  frame False {
                  }
                  frame True {
                    "Confocal Y 2 (V)" <- w3198
                    "Confocal X 2 (V)" <- w3197
                  }
                }
                n2215 = Or(x="Set X Only", y="Set Confocal Spot (X-Y)") -> (x .or. y?=w3170:bool)
                n2216 = Or(x="Set Confocal Spot (X-Y)", y="Set Y Only") -> (x .or. y?=w3169:bool)
                n2217 = case shown="True" w3170 {
                  tunnel: w3167 -> [_ w3199]
                  frame False {
                  }
                  frame True {
                    n2218 = property on="AO2" class="Slide (strict)"("Val(Sgnl)"=w3199) -> ()  [unwired: 2 in, 2 out]
                    "Confocal X 1 (V)" <- w3199
                  }
                }
                n2219 = case shown="True" w3169 {
                  tunnel: w3166 -> [_ w3200]
                  frame False {
                  }
                  frame True {
                    n2220 = property on="AO1" class="Slide (strict)"("Val(Sgnl)"=w3200) -> ()  [unwired: 2 in, 2 out]
                    "Confocal Y 1 (V)" <- w3200
                  }
                }
                n2221 = local write "Set High F Confocal Spot (X-Y)"(w3165) -> ()
                n2222 = local write "Set Confocal Spot (X-Y)"(w3165) -> ()
                n2223 = local write "Set X Only"(w3165) -> ()
                n2224 = local write "Set Y Only"(w3165) -> ()
              }
            }
          }
          frame 3 {
            n2225 = local read "BD 2 Frequency 1 (MHz)"() -> (w3201:dbl)
            n2226 = local read "BD 1 Frequency 1 (MHz)"() -> (w3202:dbl)
            n2227 = local write "Manipulating Trap"(TRUE ("Manipulating Trap")) -> ()
            n2228 = local write "Coords"(T7 {"Horizontal"=0, "Vertical"=0} ("Coords")) -> ()
            n2229 = while {
              tunnel: w3207 -> [w3212]
              tunnel: w3205 -> [w3211]
              tunnel: w3203 -> [w3210]
              tunnel: w3202 -> [w3209]
              tunnel: w3201 -> [w3208]
              stop <- w3213 stop-if-true
              n2230 = event shown="[0] \"Pane\": Mouse Move" {
                selector: _ -> [_ _]
                dyn-events: _ -> [_ _]
                timeout: _ -> [_ _]
                tunnel: ["Force Manip Abort" w3277] -> w3213
                tunnel: w3212 -> [w3220 _]
                tunnel: w3211 -> [w3218 _]
                tunnel: w3210 -> [w3217 _]
                tunnel: w3209 -> [w3216 _]
                tunnel: w3208 -> [w3215 _]
                event Mouse Move {
                  n2231 = event-data() -> ("Time"=w3221:u32, "Coords"=w3222:T7)  [unwired: 3 out]
                  n2232 = Less?(x=w3221, y=w3220) -> (x < y?=w3219:bool)
                  n2233 = case "Makes sure old motion events prior to mouse click aren't used" shown="False" w3219 {
                    tunnel: w3222 -> [w3264 _]
                    tunnel: w3218 -> [w3265 _]
                    tunnel: w3217 -> [w3242 _]
                    tunnel: w3216 -> [w3238 _]
                    tunnel: w3215 -> [w3237 _]
                    frame False {
                      n2234 = Subtract(x=w3264, y=w3265) -> (x-y=w3263:T7)
                      "Coords" <- w3263
                      n2235 = local read "Y RF Frequency Limits (MHz)"() -> (w3223:T17)
                      n2236 = To Double Precision Float(number=w3263) -> (double precision float=w3262:cluster{"Horizontal":dbl, "Vertical":dbl})
                      n2237 = Multiply(x=cluster{"Horizontal":dbl, "Vertical":dbl} {"Horizontal"=-1.0, "Vertical"=1.0}, y="Manipulation Scaling") -> (x*y=w3258:cluster{"Horizontal":dbl, "Vertical":dbl})
                      n2238 = local read "X RF Frequency Limits (MHz)"() -> (w3224:T17)
                      n2239 = Multiply(x=w3262, y=w3258) -> (x*y=w3260:cluster{"Horizontal":dbl, "Vertical":dbl})
                      n2240 = Unbundle By Name(w3260) -> ("Horizontal"=w3255:dbl, "Vertical"=w3259:dbl)
                      n2241 = Unbundle By Name(w3223) -> ("Maximum"=w3226:dbl, "Minimum"=w3225:dbl)
                      n2242 = Boolean To (0,1)(Boolean="Manip. X?") -> (0, 1=w3253:i16)
                      n2243 = Boolean To (0,1)(Boolean="Manip. Y?") -> (0, 1=w3250:i16)
                      n2244 = local read "BD 1 Frequency 2 (MHz)"() -> (w3240:dbl)
                      n2245 = Multiply(x=w3259, y=w3250) -> (x*y=w3252:dbl)
                      n2246 = Multiply(x=w3253, y=w3255) -> (x*y=w3256:dbl)
                      n2247 = local read "BD 2 Frequency 2 (MHz)"() -> (w3239:dbl)
                      n2248 = Unbundle By Name(w3224) -> ("Maximum"=w3228:dbl, "Minimum"=w3227:dbl)
                      n2249 = Add(x=w3237, y=w3252) -> (x+y=w3230:dbl)
                      n2250 = Add(x=w3238, y=w3256) -> (x+y=w3232:dbl)
                      n2251 = In Range and Coerce(upper limit=w3228, x=w3232, lower limit=w3227) -> (coerced(x)=w3231:dbl)  [unwired: 1 out]
                      n2252 = In Range and Coerce(upper limit=w3226, x=w3230, lower limit=w3225) -> (coerced(x)=w3229:dbl)  [unwired: 1 out]
                      n2253 = Subtract(x=w3231, y=w3240) -> (x-y=w3249:dbl)
                      n2254 = Subtract(x=w3229, y=w3239) -> (x-y=w3248:dbl)
                      n2255 = Square(x=w3249) -> (x^2=w3247:dbl)
                      n2256 = Square(x=w3248) -> (x^2=w3246:dbl)
                      n2257 = Add(x=w3247, y=w3246) -> (x+y=w3245:dbl)
                      n2258 = Square Root(x=w3245) -> (sqrt(x)=w3241:dbl)
                      n2259 = In Range and Coerce(upper limit="Limit Max (MHz)", x=w3241, lower limit="Limit Min (MHz)") -> (In Range?=w3234:bool)  [unwired: 1 out]
                      n2260 = Not(x="Limits Enable") -> (.not. x?=w3233:bool)
                      n2261 = Or(x=w3234, y=w3233) -> (x .or. y?=w3235:bool)
                      n2262 = case shown="True" w3235 {
                        tunnel: w3242 -> [_ w3275]
                        tunnel: w3241 -> [_ w3266]
                        tunnel: w3231 -> [_ w3273]
                        tunnel: w3240 -> [_ w3272]
                        tunnel: w3229 -> [_ w3271]
                        tunnel: w3239 -> [_ w3270]
                        tunnel: w3224 -> [_ w3268]
                        tunnel: w3223 -> [_ w3267]
                        frame False {
                        }
                        frame True {
                          n2263 = local read "BD 1 Frequency 3 (MHz)"() -> (w3274:dbl)
                          n2264 = local read "BD 2 Frequency 3 (MHz)"() -> (w3269:dbl)
                          n2265 = local write "Trap D (MHz)"(w3266) -> ()
                          n2266 = call "set RF board frequency - interlace.vi"("Board 2 Frequency Limits"=w3267, "Board 1 Frequency Limits"=w3268, "FPGA VI Reference In"=w3275, "Board 2 Frequency 3 (MHz)"=w3269, "Board 1 Frequency 3 (MHz)"=w3274, "Board 2 Frequency 2 (MHz)"=w3270, "Board 2 Frequency 1 (MHz)"=w3271, "Board 1 Frequency 2 (MHz)"=w3272, "Board 1 Frequency 1  (MHz)"=w3273) -> ()  [unwired: 1 in, 2 out]
                          n2267 = local write "BD 2 Frequency 1 (MHz)"(w3271) -> ()
                          n2268 = local write "BD 1 Frequency 1 (MHz)"(w3273) -> ()
                        }
                      }
                    }
                    frame True {
                    }
                  }
                }
                event Mouse Up {
                  n2269 = event-data() -> ("Button"=w3276:u16)  [unwired: 8 out]
                  n2270 = case shown="3" w3276 {
                    tunnel: [FALSE TRUE] -> w3277
                    frame 0, Default {
                    }
                    frame 3 {
                      n2271 = local read "Trap D (MHz)"() -> (w3279:dbl)
                      n2272 = property on="Initial D (MHz)" class="DigNum (strict)"("Val(Sgnl)"=w3279) -> ()  [unwired: 2 in, 2 out]
                      n2273 = local write "Manipulating Trap"(FALSE ("Manipulating Trap")) -> ()
                    }
                  }
                }
              }
            }
          }
        }
      }
      event Mouse Move {
        n2274 = event-data() -> ()  [unwired: 6 out]
      }
    }
    n2275 = local read "Stop All"() -> (w3062:bool)
    n2276 = node-c288() -> ()  [unwired: 2 out]
  }
  n2277 = node-c288(w119) -> ()  [unwired: 1 out]
  n2278 = node-c288(w121) -> ()  [unwired: 1 out]
  n2279 = node-c288(w107) -> ()  [unwired: 1 out]
  n2280 = flat-sequence "Video" {
    tunnel: [w3290] -> w109
    tunnel: w109 -> [w3331]
    frame #0 {
      n2281 = while {
        stop <- w3283 continue-if-true
        n2282 = call "Close Video Capture.vi"() -> ("error code OUT"=w3285:i32)
        n2283 = Equal?(x=w3285, y=0) -> (x = y?=w3283:bool)
      }
      n2284 = local write "Stop All"(FALSE ("Stop All")) -> ()
    }
    frame #1 {
      n2285 = call "DMR_Init.vi"() -> ()  [unwired: 3 out]
    }
    frame #2 {
      # "Setting the destination format to Mono8 makes sure that the image can be displayed in the intensity plot."
      n2286 = call "DMR_GetDevice.vi"("search string IN"="DE019116701") -> ("device handle OUT"=w3308:i32)  [unwired: 4 in, 2 out]
      n2287 = call "DMR_OpenDevice.vi"("device handle IN"=w3308) -> ("driver handle OUT"=w3291:i32)  [unwired: 4 out]
      n2288 = call "DMR_FindList.vi"("flags IN"=u32 0 ("flags"), "list name IN"="" ("String"), "list type IN"=T33."camera descriptions", "driver handle IN"=w3291) -> ("list handle OUT"=w3294:i32)  [unwired: 2 out]
      n2289 = call "DMR_FindList.vi"("flags IN"=u32 0 ("flags"), "list name IN"="Base", "list type IN"=T33."setting", "driver handle IN"=w3291) -> ("list handle OUT"=w3292:i32)  [unwired: 2 out]
      n2290 = call "OBJ_GetHandle.vi"("object name IN"="VideoStandard", "list handle IN"=w3294) -> ("object handle OUT"=w3288:i32)  [unwired: 3 out]
      n2291 = call "OBJ_GetHandle.vi"("object name IN"="PixelFormat", "list handle IN"=w3292) -> ("object handle OUT"=w3302:i32)  [unwired: 3 out]
      n2292 = call "OBJ_SetS.vi"("value index IN"=0, "value IN"="NTSC M", "object handle IN"=w3288) -> ()  [unwired: 2 out]
      n2293 = call "OBJ_SetS.vi"("value index IN"=0, "value IN"="Mono8" ("value"), "object handle IN"=w3302) -> ()  [unwired: 2 out]
      n2294 = call "OBJ_GetHandle.vi"("object name IN"="VideoChannel", "list handle IN"=w3292) -> ("object handle OUT"=w3298:i32)  [unwired: 3 out]
      n2295 = while {
        tunnel: [w3313] -> w3290
        tunnel: w3291 -> [w3310]
        stop <- w3311 continue-if-true
        n2296 = call "DMR_ImageRequestSingle.vi"("request control IN"=0, "driver handle IN"=w3310) -> ("error code OUT"=w3312:i32, "driver handle OUT"=w3313:i32)  [unwired: 2 out]
        n2297 = Equal To 0?(x=w3312) -> (x = 0?=w3311:bool)
      }
      n2298 = call "OBJ_SetI.vi"("value index IN"=0, "value IN"=3 ("Video channel"), "object handle IN"=w3298) -> ()  [unwired: 2 out]
    }
    frame #3 {
      w3319 = T18 0 items=["Grayscale (U8)", "Grayscale (I16)", "Grayscale (SGL)", "Complex (CSG)", "RGB (U32)", "HSL (U32)", "RGB (U64)"] ("Image Type")
      w3327 = T18 0 items=["Grayscale (U8)", "Grayscale (I16)", "Grayscale (SGL)", "Complex (CSG)", "RGB (U32)", "HSL (U32)", "RGB (U64)"] ("Image Type")
      n2299 = for "Create Greyscale map" {
        N: 256 -> [_]
        tunnel: [w3333] -> w3316 mode=indexing
        workers-P: _ -> [_]
        i -> [w3336]
        n2300 = To Unsigned Byte Integer(number=w3336) -> (unsigned 8bit integer=w3332:u8)
        n2301 = Join Numbers(hi=w3332, lo=w3332) -> ((hi.lo)=w3335:u16)
        n2302 = Join Numbers(hi=w3332, lo=w3332) -> ((hi.lo)=w3334:u16)
        n2303 = Join Numbers(hi=w3335, lo=w3334) -> ((hi.lo)=w3333:u32)
      }
      n2304 = call "IMAQ Create"("Image Name"="Scaled video", "Image Type"=w3319) -> ("New Image"=w3318:T2)  [unwired: 2 in, 2 out]
      n2305 = call "IMAQ Create"("Image Name"="Main video", "Image Type"=w3327) -> ("New Image"=w3328:T2)  [unwired: 2 in, 2 out]
      n2306 = node-c288(0 ("Processor")) -> (w3326:T22)  [unwired: 3 out]
      n2307 = Initialize Array(u32 0 ("Window Number (0...15)"), 480 ("dimension size"), 640 ("dimension size")) -> (w3321:u32[][])
      n2308 = timed-loop {
        tunnel: w3331 -> [w3353]
        tunnel: [w3352] -> w3330
        tunnel: w3328 -> [w3351]
        timing: w3326 -> [_]
        timing-out: [_] -> w3325
        tunnel: w3321 -> [w3340]
        tunnel: w3318 -> [w3338]
        tunnel: w3316 -> [w3337]
        stop <- w3339 stop-if-true
        # "This block performs the \nactual image capture."
        n2309 = node-c288() -> ()  [unwired: 2 out]
        n2310 = local read "Stop All"() -> (w3339:bool)
        n2311 = Reciprocal(x="Video Capture Rate (Hz)") -> (1/x=w3343:dbl)
        n2312 = Multiply(x=w3343, y=1000.0) -> (x*y=w3341:dbl)
        n2313 = call "DMR_ImageRequestWaitFor.vi"("queue number IN"=0, "timeout(ms) IN"=500, "driver handle IN"=w3353) -> ("error code OUT"=w3357:i32, "request number OUT"=w3354:i32, "driver handle OUT"=w3355:i32)
        n2314 = feedback #1(T34 refnum ("Avi Refnum")) -> (w3345:T34)
        n2315 = case shown="True" "New Video File" {
          tunnel: [T34 refnum ("Avi Refnum") w3374] -> w3347
          tunnel: [FALSE TRUE] -> w3348
          tunnel: w3345 -> [_ w3370]
          frame False {
          }
          frame True {
            n2316 = call "Create new save file.vi"("Ext"=".avi" ("string"), "Index In"="Video Index") -> ("Path Out"=w3366:path, "Index Out"=w3367:dbl)  [unwired: 1 in]
            "Path Out" <- w3366
            n2317 = Not Equal?(x=w3370, y=T34 refnum ("Avi Refnum")) -> (x != y?=w3371:bool)
            n2318 = Increment(x=w3367) -> (x+1=w3376:dbl)
            n2319 = case shown="True" w3371 {
              tunnel: w3370 -> [_ w3377]
              frame False {
              }
              frame True {
                n2320 = call "IMAQ AVI Close"("Avi Refnum"=w3377) -> ()  [unwired: 1 in, 10 out]
              }
            }
            n2321 = local write "Video Index"(w3376) -> ()
            n2322 = call "IMAQ AVI Create"("Frames Per Second"=u32 30, "AVI Path"=w3366) -> ("Avi Refnum"=w3374:T34)  [unwired: 5 in, 4 out]
          }
        }
        n2323 = Equal To 0?(x=w3357) -> (x = 0?=w3356:bool)
        n2324 = Select(t=w3347, s=w3348, f=w3345) -> (s? t:f=w3346:T34)
        n2325 = feedback-in #1(w3346) -> ()
        n2326 = case shown="True" w3356 {
          tunnel: w3355 -> [w3378 w3405]
          tunnel: w3354 -> [_ w3404]
          tunnel: [w3378 w3401] -> w3352
          tunnel: w3351 -> [_ w3382]
          tunnel: w3340 -> [_ w3389]
          tunnel: w3346 -> [_ w3387]
          tunnel: w3338 -> [_ w3383]
          tunnel: w3337 -> [_ w3384]
          frame False {
          }
          frame True {
            w3395 = u32 0 ("X-offset IN")
            n2327 = call "DMR_GetImageRequestBufferData.vi"("driver handle IN"=w3405, "request number IN"=w3404) -> ("width OUT"=w3394:i32, "height OUT"=w3393:i32, "driver handle OUT"=w3400:i32, "request number OUT"=w3399:i32, "bytes per pixel OUT"=w3396:i32)  [unwired: 13 out]
            n2328 = call "DMR_GetImageRequestBufferImageData.vi"("driver handle IN"=w3400, "request number IN"=w3399, "bytes per pixel IN"=w3396, "X-offset IN"=w3395, "Y-offset IN"=w3395, "height IN"=w3393, "width IN"=w3394) -> ("driver handle OUT"=w3398:u32, "request number OUT"=w3397:u32, "image OUT"=w3390:u32[][])  [unwired: 10 out]
            n2329 = call "DMR_ImageRequestUnlock.vi"("request number IN"=w3397, "driver handle IN"=w3398) -> ("driver handle OUT"=w3403:i32)  [unwired: 1 in, 2 out]
            n2330 = case shown="True" "Averaging" {
              tunnel: w3390 -> [w3446 w3451]
              tunnel: [w3446 w3450] -> w3386
              tunnel: w3389 -> [_ w3448]
              frame False {
              }
              frame True {
                (unwired) 1
                w3456 = 1
                n2331 = feedback #2(w3448) -> (w3447:u32[][])
                n2332 = Add(x=w3451, y=w3447) -> (x+y=w3452:u32[][])
                n2333 = Select(t=w3448, s="Reset Averaging", f=w3452) -> (s? t:f=w3454:u32[][])
                n2334 = feedback-in #2(w3454) -> ()
                n2335 = feedback #3(w3456) -> (w3449:i32)
                n2336 = Divide(x=w3452, y=w3449) -> (x/y=w3453:dbl[][])
                n2337 = Increment(x=w3449) -> (x+1=w3457:i32)
                n2338 = To Unsigned Long Integer(number=w3453) -> (unsigned 32bit integer=w3450:u32[][])
                n2339 = Select(t=w3456, s="Reset Averaging", f=w3457) -> (s? t:f=w3455:i32)
                n2340 = feedback-in #3(w3455) -> ()
              }
            }
            n2341 = call "DMR_ImageRequestSingle.vi"("request control IN"=0, "driver handle IN"=w3403) -> ("driver handle OUT"=w3401:i32)  [unwired: 3 out]
            n2342 = disable-structure shown="Disabled" {
              disable-tunnel: w3386 -> [w3423 _]
              disable-tunnel: w3383 -> [w3422 _]
              frame Disabled {
                n2343 = To Double Precision Float(number=w3423) -> (double precision float=w3421:dbl[][])
                n2344 = In Range and Coerce(upper limit="Intensity Upper", x=w3421, lower limit="Intensity Lower") -> (coerced(x)=w3420:dbl[][])  [unwired: 1 out]
                n2345 = Subtract(x="Intensity Upper", y="Intensity Lower") -> (x-y=w3417:dbl)
                n2346 = Subtract(x=w3420, y="Intensity Lower") -> (x-y=w3418:dbl[][])
                n2347 = Divide(x=w3418, y=w3417) -> (x/y=w3419:dbl[][])
                n2348 = Multiply(x=255.0, y=w3419) -> (x*y=w3415:dbl[][])
                n2349 = To Unsigned Byte Integer(number=w3415) -> (unsigned 8bit integer=w3424:u8[][])
                n2350 = call "IMAQ ArrayToImage"("Image Pixels (U8)"=w3424, "Image"=w3422) -> ("Image Out"=w3411:T2)  [unwired: 4 in, 5 out]
                n2351 = First Call?() -> (First Call?: T/F=w3412:bool)
                n2352 = case shown="True" w3412 {
                  tunnel: w3411 -> [w3425 w3436]
                  frame False {
                    n2353 = flat-sequence {
                      tunnel: w3425 -> [w3431]
                      frame #0 {
                        w3428 = FALSE ("Get/Set Status? (Set)")
                        w3427 = 0 ("Window Number (0...15)")
                        n2354 = call "IMAQ WindSize"("Get/Set Status? (Set)"=w3428, "Window Number"=w3427) -> ("Width & Height out"=→"Window Size":cluster{"Width":i32, "Height":i32})  [unwired: 4 in, 2 out]
                        n2355 = call "IMAQ WindMove"("Window Number (0...15)"=w3427, "Get/Set Status? (Set)"=w3428) -> ("Coordinates (screen)"=→"Window Position":cluster{"X Position":i32, "Y Position":i32})  [unwired: 3 in, 1 out]
                        n2356 = call "IMAQ WindDraw"("Resize to Image Size? (Y)"=FALSE, "Window Number (0...15)"=w3427, "Image"=w3431) -> ()  [unwired: 7 in, 2 out]
                      }
                      frame #1 {
                        n2357 = call "IMAQ WindZoom 2"("Center Point"="Center Point", "Zoom to Fit? (False)"=FALSE, "Zoom Factor"="Zoom Factor") -> ()  [unwired: 5 in, 4 out]
                      }
                    }
